vi "Reportes.vi"() -> ()   [LabVIEW 2012]
uses:
  <vilib>/addons/database/Auxilliary.llb/DB Tools Cursor Type.ctl
  <vilib>/addons/database/Connection.llb/DB Tools Open Connec (Path).vi
  <vilib>/addons/database/Connection.llb/Conn Execute.vi
  <vilib>/addons/database/Recordset.llb/Rec Fetch String Data (R).vi
  <vilib>/addons/database/Recordset.llb/Rec Destroy - Connection.vi
  <vilib>/addons/database/Recordset.llb/Rec Fetch Recordset Data (R).vi
  <vilib>/addons/database/_DB Variant To Data/Database Variant To Data.xnode
  <vilib>/addons/database/NI_Database_API.lvlib
panel:
  in  "Orden":bool
  in  "Fecha Inicial":timestamp format="%<%d/%m/%y>T"
  in  "Fecha Final":timestamp format="%<%d/%m/%y>T"
  in  "Fechas":bool
  in  "Evento":u16(ring) items=["TODOS", "Falta Producto", "Máquina Abierta", "Máquina Cerrada", "Servicio Técnico", "Automático"]
  in  "POC":u16(ring) items=["TODOS", "POC 0", "POC 1", "POC 2"]
  out "Data":string[][](table)
  in  "stop":bool
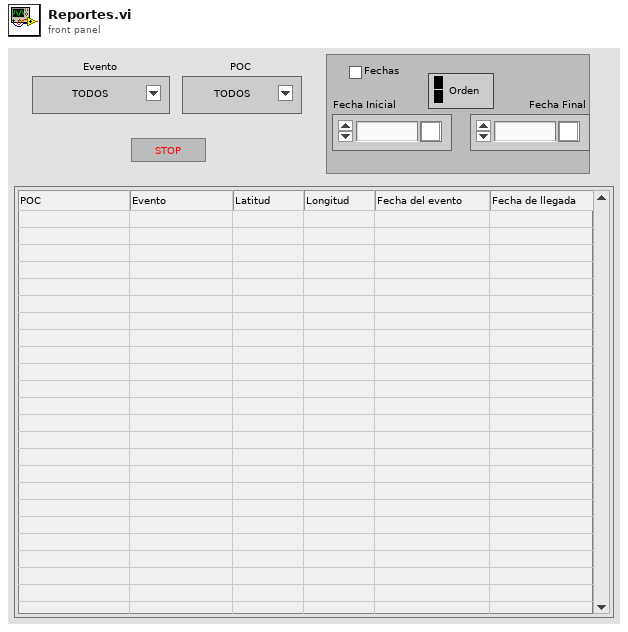
[diagram p1: front panel]
types:
  T1 = typedef "NI_Database_API.lvlib/Conn ObjectReference.ctl" = refnum<k1>
  T2 = enum16{"POC", "Imei", "Evento", "Lat", "Lon", "F_H_eve", "F_H_rec", "AVL_N", "AVL_pass", "Propietario", "Razon_Social", "Direccion", "Propietario_N", "Ciudad", "Marca", "Ruta", "N_Ruta", "Auditor", "Auditor_N"}
  T3 = typedef "NI_Database_API.lvlib/DB Tools Cursor Type.ctl" = enum16{"forward-only", "keyset", "dynamic", "static"}
  T4 = typedef "NI_Database_API.lvlib/Rec ObjectReference.ctl" = refnum<k1>
  T5 = typedef "LVDateTimeRec.ctl" = cluster{"fractional second":dbl, "second":i32, "minute":i32, "hour":i32, "day of month":i32, "month":i32, "year":i32, "day of week":i32, "day of year":i32, "DST":i32}
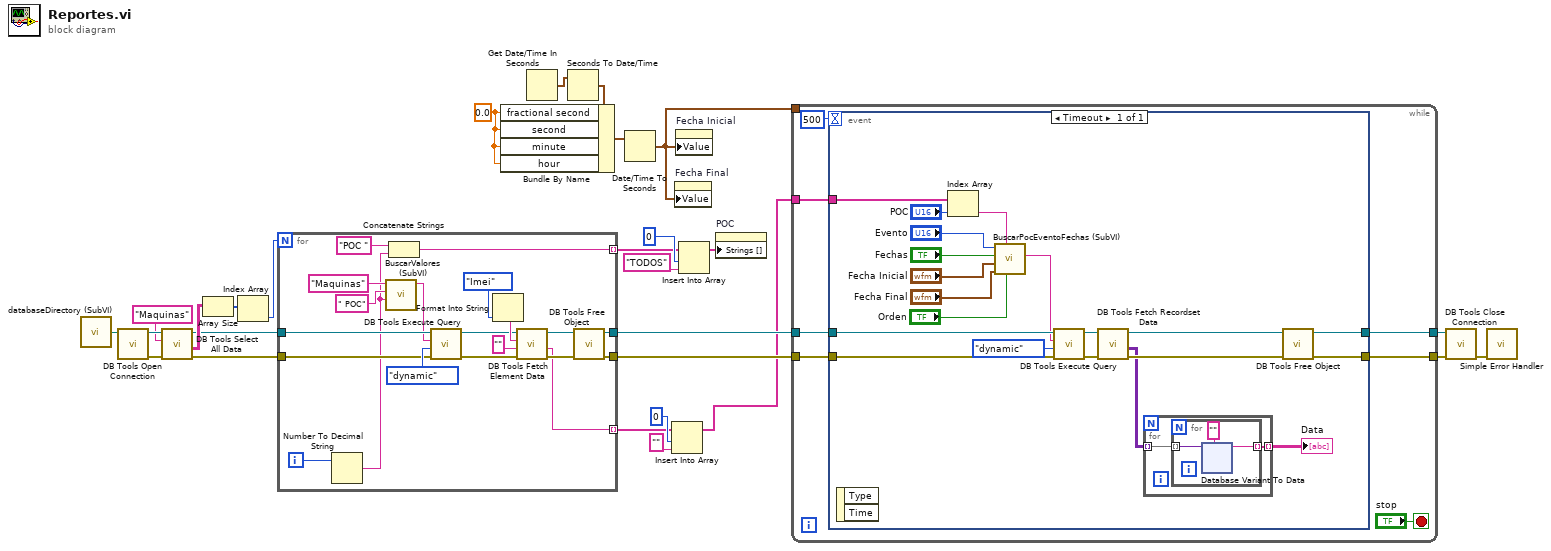
[diagram p0: block diagram]
diagram:
  w2 = 0.0 ("fractional second")
  n1 = call "databaseDirectory (SubVI).vi"() -> ("Application Directory"=w14:path)  [unwired: 1 in]
  n2 = call-poly <vilib>:"DB Tools Open Connection.vi"("connection information"=w14) -> ("error out"=w19:errorcluster, "connection reference"=w18:T1)  [unwired: 7 in]
  n3 = call <vilib>:"DB Tools Select All Data.vi"("error in (no error)"=w19, "table"="Maquinas", "connection reference"=w18) -> ("error out"=w13:errorcluster, "data"=w21:string[][], "connection reference out"=w17:T1)  [unwired: 3 in]
  n4 = Array Size(array=w21) -> (size(s)=w20:i32[])
  n5 = Index Array(array=w20) -> (element=w15:i32)  [unwired: 1 in]
  n6 = for {
    N: w15 -> [_]
    tunnel: w17 -> [w42]
    tunnel: w13 -> [w43]
    tunnel: [w41] -> w11
    tunnel: [w40] -> w10
    tunnel: [w30] -> w12 mode=indexing
    tunnel: [w29] -> w7 mode=indexing
    i -> [w28]
    n7 = Number To Decimal String(number=w28) -> (decimal integer string=w32:string)  [unwired: 1 in]
    n8 = call "BuscarValores (SubVI).vi"("="=w32, "Columna"=" POC" ("Substring"), "Tabla"="Maquinas" ("table")) -> ("String"=w39:string)  [unwired: 8 in]
    n9 = Concatenate Strings("POC " ("string"), w32) -> (w30:string)
    n10 = call-poly <vilib>:"DB Tools Execute Query.vi"("error in (no error)"=w43, "cursor type"=DB_Tools_Cursor_Type."dynamic", "SQL query"=w39, "connection reference"=w42) -> ("error out"=w35:errorcluster, "recordset reference"=w36:T4)  [unwired: 4 in]
    n11 = Format Into String(T2."Imei") -> (resulting string=w47:string)  [unwired: 3 in, 1 out]
    n12 = call-poly <vilib>:"DB Tools Fetch Element Data.vi"("error in (no error)"=w35, "type"="", "column index"=w47, "recordset reference"=w36) -> ("error out"=w33:errorcluster, "data"=w29:string, "recordset reference out"=w34:T4)  [unwired: 3 in]
    n13 = call-poly <vilib>:"DB Tools Free Object.vi"("error in (no error)"=w33, "recordset reference"=w34) -> ("error out"=w40:errorcluster, "connection reference"=w41:T1)  [unwired: 8 in]
  }
  n14 = Get Date/Time In Seconds() -> (seconds since 1Jan1904=w5:timestamp)
  n15 = Seconds To Date/Time(time stamp (now)=w5) -> (date time rec=w4:T5)  [unwired: 1 in]
  n16 = Bundle By Name(cluster=w4, "fractional second"=w2, "second"=w2, "minute"=w2, "hour"=w2) -> (w3:T5)
  n17 = Date/Time To Seconds(2:w3) -> (0:w1:timestamp)  [unwired: 1 in]
  n18 = Insert Into Array(array=w7, index=0, new element="" ("new element/subarray")) -> (w6:string[])
  n19 = property on="Fecha Final" class="AbsTime (strict)"("Value"=w1) -> ()  [unwired: 2 in, 2 out]
  n20 = property on="Fecha Inicial" class="AbsTime (strict)"("Value"=w1) -> ()  [unwired: 2 in, 2 out]
  n21 = Insert Into Array(array=w12, index=0, new element="TODOS" ("new element/subarray")) -> (w22:string[])
  n22 = property on="POC" class="Ring (strict)"("Strings []"=w22) -> ()  [unwired: 2 in, 2 out]
  n23 = while {
    tunnel: w11 -> [w54]
    tunnel: w10 -> [w53]
    tunnel: [w51] -> w26
    tunnel: [w50] -> w25
    tunnel: w6 -> [w48]
    tunnel: w1 -> [_]
    stop <- "stop" stop-if-true
    n24 = event shown="[0] Timeout" {
      selector: _ -> [_]
      dyn-events: _ -> [_]
      timeout: 500 -> [_]
      tunnel: w54 -> [w72]
      tunnel: w53 -> [w71]
      tunnel: [w68] -> w51
      tunnel: [w67] -> w50
      tunnel: w48 -> [w58]
      event Timeout {
        n25 = event-data() -> ()  [unwired: 1 in, 2 out]
        n26 = Index Array(array=w58, index="POC") -> (element=w57:string)
        n27 = call "BuscarPocEventoFechas (SubVI).vi"("Orden"="Orden", "Imei"=w57, "Fecha Final"="Fecha Final", "Fecha Inicial"="Fecha Inicial", "Fechas"="Fechas", "Evento"="Evento") -> ("Query"=w61:string)  [unwired: 5 in]
        n28 = call-poly <vilib>:"DB Tools Execute Query.vi"("error in (no error)"=w71, "cursor type"=DB_Tools_Cursor_Type."dynamic", "SQL query"=w61, "connection reference"=w72) -> ("error out"=w73:errorcluster, "recordset reference"=w74:T4)  [unwired: 4 in]
        n29 = call-poly <vilib>:"DB Tools Fetch Recordset Data.vi"("error in (no error)"=w73, "recordset reference"=w74) -> ("error out"=w69:errorcluster, "recordset data"=w66:variant[][], "recordset reference out"=w70:T4)  [unwired: 3 in]
        n30 = for {
          tunnel: w66 -> [w76] mode=indexing
          tunnel: [w75] -> w60 mode=indexing
          n31 = for {
            tunnel: w76 -> [w78] mode=indexing
            tunnel: [w77] -> w75 mode=indexing
            n32 = xnode "Database Variant To Data"("database variant"=w78, "type"="") -> ("data"=w77:string)  [unwired: 1 in, 1 out]
          }
        }
        "Data" <- w60
        n33 = call-poly <vilib>:"DB Tools Free Object.vi"("error in (no error)"=w69, "recordset reference"=w70) -> ("error out"=w67:errorcluster, "connection reference"=w68:T1)  [unwired: 8 in]
      }
    }
  }
  n34 = call <vilib>:"DB Tools Close Connection.vi"("error in (no error)"=w25, "connection reference"=w26) -> ("error out"=w27:errorcluster)  [unwired: 5 in]
  n35 = call <vilib>:"Simple Error Handler.vi"("error in (no error)"=w27) -> ()  [unwired: 4 in, 5 out]
